vi "bk9201 Read.vi"(11 "VISA resource name":refnum<visa-resource-name>="USB0::0xFFFF::0x9200::802243020766810010::INSTR") -> (0 "error out":errorcluster, 1 "Actual Power":dbl format="%.4g", 2 "Actual Current":dbl format="%.4g", 3 "Actual Voltage":dbl format="%.4g")   [LabVIEW 2018]
uses:
  <instrlib>/BK Precision 9200 Series/BK Precision 9200 Series.lvlib
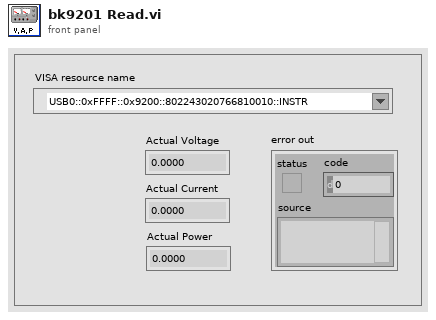
[diagram p1: front panel]
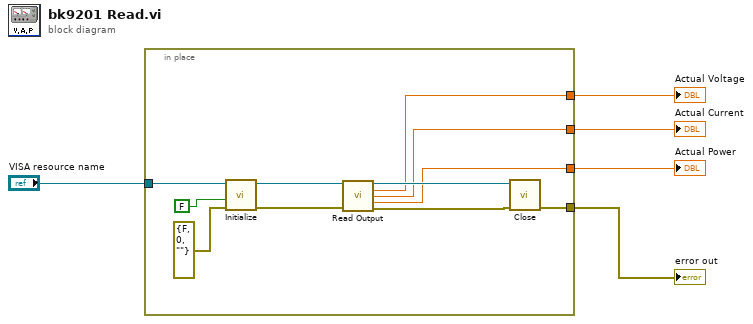
[diagram p0: block diagram]
diagram:
  n1 = in-place {
    in-place-border: "VISA resource name" -> [w16]
    in-place-border: [w13] -> w4
    in-place-border: [w12] -> w3
    in-place-border: [w11] -> w2
    in-place-border: [w10] -> w1
    n2 = call <instrlib>:"Initialize.vi"("error in (no error)"=errorcluster {"status"=FALSE, "code"=0, "source"=""}, "Reset (True)"=FALSE, "VISA resource name"=w16) -> ("error out"=w8:errorcluster, "VISA resource name out"=w15:refnum<visa-resource-name>)  [unwired: 7 in]
    n3 = call <instrlib>:"Read Output.vi"("VISA resource name"=w15, "error in (no error)"=w8) -> ("VISA resource name out"=w14:refnum<visa-resource-name>, "Actual Voltage Level (V)"=w12:dbl, "Actual Current Level (A)"=w11:dbl, "Actual Power Level (W)"=w10:dbl, "error out"=w9:errorcluster)  [unwired: 9 in]
    n4 = call <instrlib>:"Close.vi"("error in (no error)"=w9, "VISA resource name"=w14) -> ("error out"=w13:errorcluster)  [unwired: 9 in]
  }
  "error out" <- w4
  "Actual Voltage" <- w3
  "Actual Current" <- w2
  "Actual Power" <- w1
